vi "EXCOM_CRASH_TEST.vi"() -> ()   [LabVIEW 2011]
panel:
  in  "Infinite":bool
  out "TCP_string":string
  in  "offset DEC":dbl
  in  "offset RA":dbl
  in  "DEC (fix)":dbl format="%<%H:%M:%S%1u>t"
  in  "HA (fix)":dbl format="%<%H:%M:%S%1u>t"
  out "HA 2":dbl format="%.2f"
  out "DEC 2":dbl format="%.2f"
  out "NODEC":dbl format="%<%H:%M:%S%0u>t"
  out "NORA":dbl format="%<%H:%M:%S%1u>t"
  out "Epoque":dbl format="%.2f"
  out "DEC":dbl format="%<%H:%M:%S>t"
  out "RA":dbl format="%<%H:%M:%S%1u>t"
  out "HA":dbl format="%<%H:%M:%S%1u>t"
  out "Année":dbl format="%.2f"
  in  "Ring":u16(ring) items=["0 - No Command"=0, "1 - Update time and date"=1, "2 - ZDOMECOMMAND"=2, "3 - ZPOINT"=3, "4 - ZROTATOR"=4, "5 - ZFOCUS"=5, "6 - SLEW"=6, "7 - OFFSET"=7, "8 - OBJECT"=8, "9 - TMOVE"=9, "10 - ZENITH"=10, "11 - START TRAIL"=11, "12 - GO"=12, "13 - STOP"=13, "22 - DOEPOCH"=22, "36 - HA DEC SLEW"=36]
  out "STATLH":bool[](array[boolean])
  out "STATEX":bool[](array[boolean])
  in  "Délai de communication":u32(knob) scale=5.0..5000.0
  out "STATH":bool[](array[boolean])=[FALSE, FALSE, TRUE, TRUE, FALSE, TRUE, TRUE, FALSE, FALSE, FALSE, FALSE, FALSE, FALSE, FALSE, FALSE, FALSE, FALSE, FALSE, FALSE, FALSE, FALSE, FALSE, FALSE, FALSE, FALSE, FALSE, FALSE, FALSE, FALSE, FALSE, FALSE, FALSE]
  out "STATL":bool[](array[boolean])=[TRUE, FALSE, FALSE, FALSE, FALSE, FALSE, FALSE, FALSE, FALSE, FALSE, FALSE, FALSE, FALSE, FALSE, FALSE, FALSE, FALSE, FALSE, FALSE, FALSE, FALSE, FALSE, FALSE, FALSE, FALSE, FALSE, FALSE, FALSE, FALSE, FALSE, FALSE, FALSE]
  out "error out":errorcluster
  in  "QUITTER":bool
  out "connection ID":refnum<k5>
  # "."
  # "HA DEC ARGS"
  # "OFFSET ARGS"
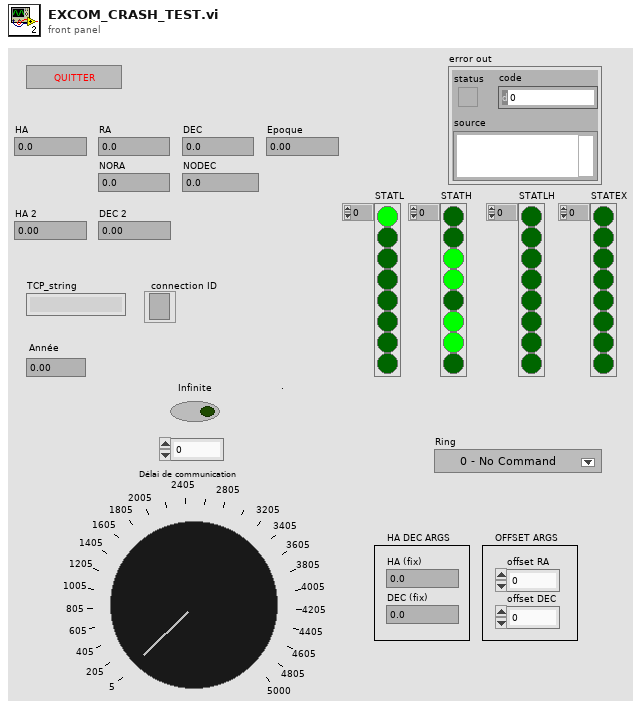
[diagram p1: front panel]
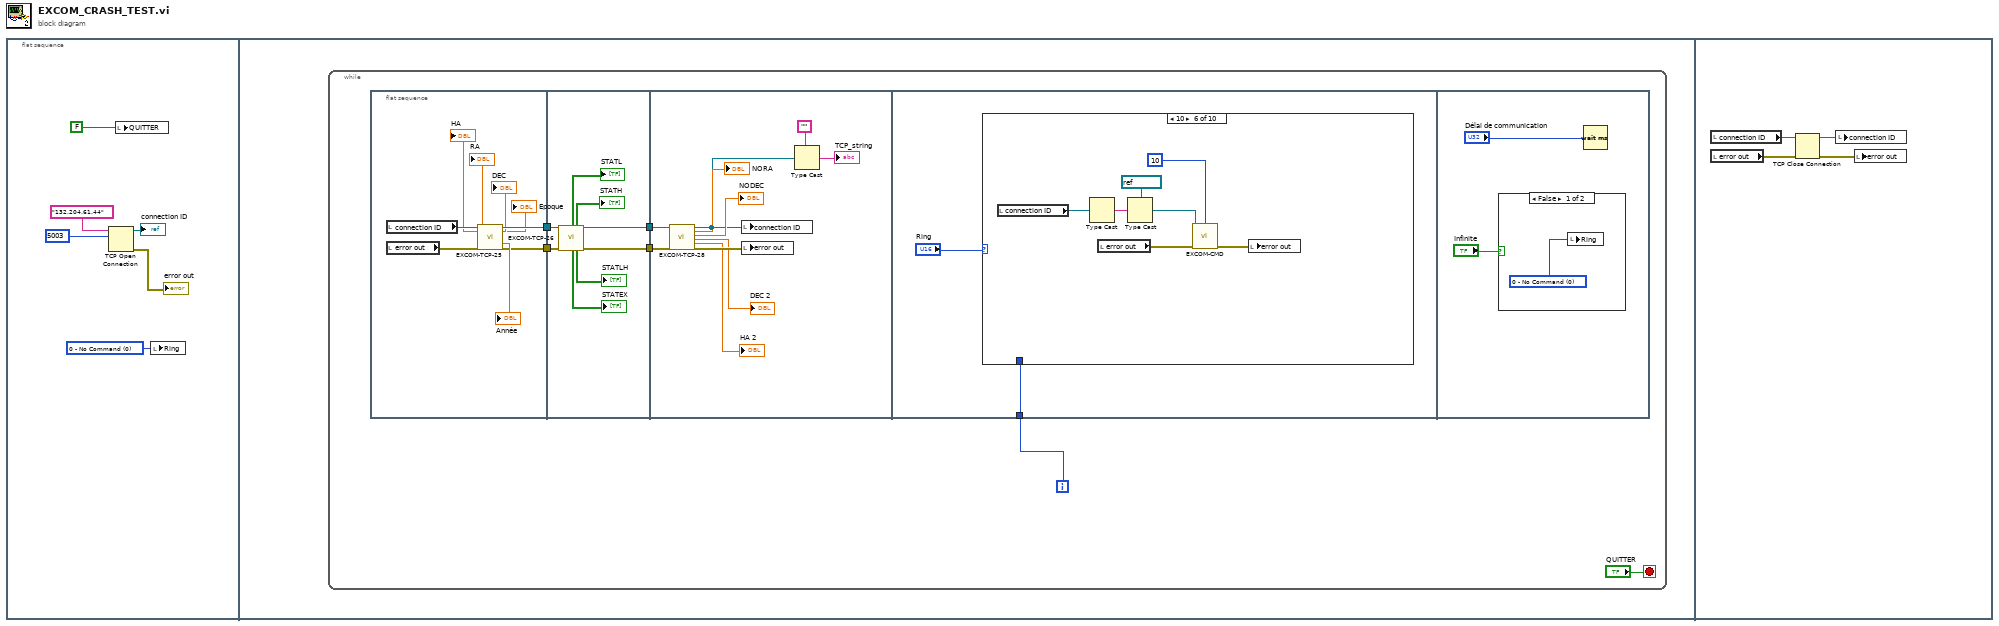
[diagram p0: block diagram]
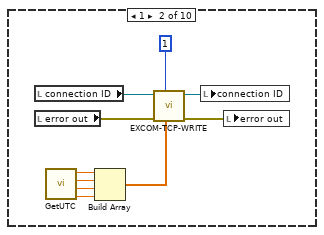
[diagram p3: hidden frame]
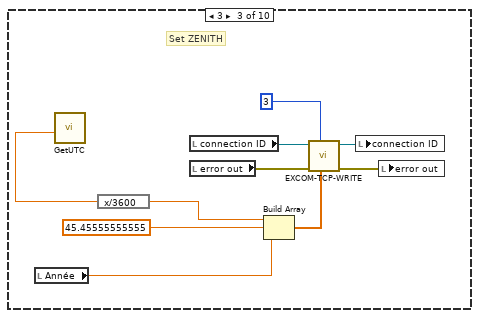
[diagram p4: hidden frame]
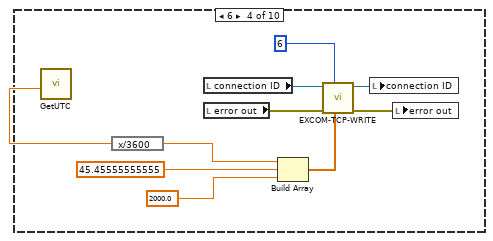
[diagram p5: hidden frame]
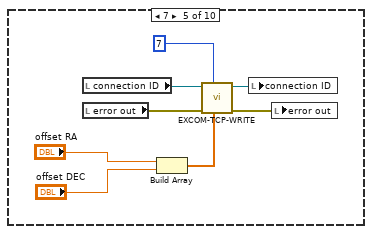
[diagram p6: hidden frame]
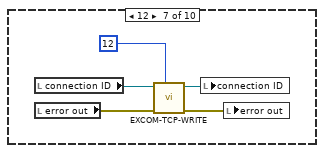
[diagram p7: hidden frame]
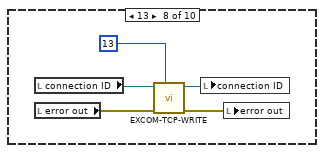
[diagram p8: hidden frame]
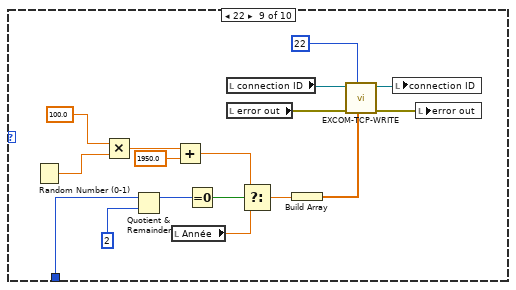
[diagram p9: hidden frame]
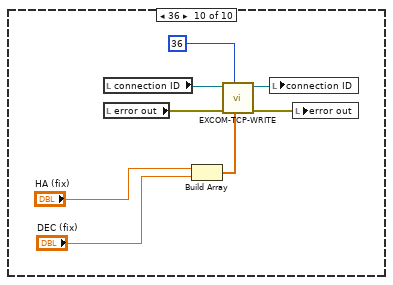
[diagram p10: hidden frame]
diagram:
  n1 = flat-sequence {
    frame #0 {
      w1 = u16 0 items=["0 - No Command"=0, "1 - Update time and date"=1, "2 - ZDOMECOMMAND"=2, "3 - ZPOINT"=3, "4 - ZROTATOR"=4, "5 - ZFOCUS"=5, "6 - SLEW"=6, "7 - OFFSET"=7, "8 - OBJECT"=8, "9 - TMOVE"=9, "10 - ZENITH"=10, "11 - START TRAIL"=11, "12 - GO"=12, "13 - STOP"=13, "22 - DOEPOCH"=22] ("Ring")
      n2 = TCP Open Connection(address="132.204.61.44", remote port or service name=u16 5003) -> (connection ID=→"connection ID":refnum<k5>, error out=→"error out":errorcluster)  [unwired: 3 in]
      n3 = local write "QUITTER"(FALSE ("QUITTER")) -> ()
      n4 = local write "Ring"(w1) -> ()
    }
    frame #1 {
      n5 = while {
        i -> [w11]
        stop <- "QUITTER" stop-if-true
        n6 = flat-sequence {
          tunnel: [w18] -> w10
          tunnel: [w17] -> w9
          tunnel: w10 -> [w24]
          tunnel: w9 -> [w25]
          tunnel: [w23] -> w8
          tunnel: [w22] -> w7
          tunnel: w8 -> [w39]
          tunnel: w7 -> [w38]
          tunnel: w11 -> [w40]
          frame #0 {
            n7 = local read "connection ID"() -> (w21:refnum<k5>)
            n8 = local read "error out"() -> (w20:errorcluster)
            n9 = call "EXCOM-TCP-25.vi"("connection ID"=w21, "Error IN"=w20) -> ("HA"=→"HA":dbl, "RA"=→"RA":dbl, "DEC"=→"DEC":dbl, "Epoque"=→"Epoque":dbl, "CID Out"=w18:refnum<k5>, "Année"=→"Année":dbl, "Error Out"=w17:errorcluster)  [unwired: 4 in, 7 out]
          }
          frame #1 {
            n10 = call "EXCOM-TCP-26.vi"("connection ID"=w24, "Error IN"=w25) -> ("STATL"=→"STATL":bool[], "STATH"=→"STATH":bool[], "CID Out"=w23:refnum<k5>, "STATEX"=→"STATEX":bool[], "STATLH"=→"STATLH":bool[], "Error Out"=w22:errorcluster)  [unwired: 8 in]
          }
          frame #2 {
            n11 = call "EXCOM-TCP-28.vi"("connection ID"=w39, "Error IN"=w38) -> ("CID Out"=w32:refnum<k5>, "NORA"=→"NORA":dbl, "NODEC"=→"NODEC":dbl, "DEC"=→"DEC 2":dbl, "HA"=→"HA 2":dbl, "Error Out"=w35:errorcluster)  [unwired: 12 in]
            n12 = local write "connection ID"(w32) -> ()
            n13 = local write "error out"(w35) -> ()
            n14 = Type Cast(type="", x=w32) -> (*(type *) &x=→"TCP_string":string)
          }
          frame #3 {
            n15 = case shown="10" "Ring" {
              tunnel: w40 -> [_ _ _ _ _ _ _ _ w103 _]
              frame 0, Default {
              }
              frame 1 {
                n16 = local read "connection ID"() -> (w51:refnum<k5>)
                n17 = local read "error out"() -> (w48:errorcluster)
                n18 = call "GetUTC.vi"() -> ("UTC_fractional"=w43:dbl, "Day"=w44:dbl, "Month"=w45:dbl, "Year"=w46:dbl)  [unwired: 5 out]
                n19 = Build Array(w46, w45, w44, w43) -> (w42:dbl[])
                n20 = call "EXCOM-TCP-WRITE.vi"("Args"=w42, "Commande #"=1, "Error IN"=w48, "connection ID"=w51) -> ("Error OUT"=w49:errorcluster, "connection ID out"=w50:refnum<k5>)  [unwired: 3 in, 2 out]
                n21 = local write "connection ID"(w50) -> ()
                n22 = local write "error out"(w49) -> ()
              }
              frame 3 {
                # "Set ZENITH"
                n23 = local read "Année"() -> (w52:dbl)
                n24 = call "GetUTC.vi"() -> ("LST+_seconds"=w53:dbl)  [unwired: 8 out]
                n25 = expression code="x/3600"(w53) -> (w55:dbl)
                n26 = local read "connection ID"() -> (w60:refnum<k5>)
                n27 = local read "error out"() -> (w57:errorcluster)
                n28 = Build Array(w55, 45.45555555555 ("element"), w52) -> (w56:dbl[])
                n29 = call "EXCOM-TCP-WRITE.vi"("Args"=w56, "Commande #"=3, "Error IN"=w57, "connection ID"=w60) -> ("Error OUT"=w58:errorcluster, "connection ID out"=w59:refnum<k5>)  [unwired: 3 in, 2 out]
                n30 = local write "connection ID"(w59) -> ()
                n31 = local write "error out"(w58) -> ()
              }
              frame 6 {
                n32 = call "GetUTC.vi"() -> ("LST+_seconds"=w63:dbl)  [unwired: 8 out]
                n33 = expression code="x/3600"(w63) -> (w64:dbl)
                n34 = local read "connection ID"() -> (w70:refnum<k5>)
                n35 = local read "error out"() -> (w67:errorcluster)
                n36 = Build Array(w64, 45.45555555555 ("element"), 2000.0 ("t")) -> (w66:dbl[])
                n37 = call "EXCOM-TCP-WRITE.vi"("Args"=w66, "Commande #"=6, "Error IN"=w67, "connection ID"=w70) -> ("Error OUT"=w68:errorcluster, "connection ID out"=w69:refnum<k5>)  [unwired: 3 in, 2 out]
                n38 = local write "connection ID"(w69) -> ()
                n39 = local write "error out"(w68) -> ()
              }
              frame 7 {
                n40 = local read "connection ID"() -> (w78:refnum<k5>)
                n41 = local read "error out"() -> (w75:errorcluster)
                n42 = Build Array("offset RA", "offset DEC") -> (w74:dbl[])
                n43 = call "EXCOM-TCP-WRITE.vi"("Args"=w74, "Commande #"=7, "Error IN"=w75, "connection ID"=w78) -> ("Error OUT"=w76:errorcluster, "connection ID out"=w77:refnum<k5>)  [unwired: 3 in, 2 out]
                n44 = local write "connection ID"(w77) -> ()
                n45 = local write "error out"(w76) -> ()
              }
              frame 10 {
                n46 = local read "connection ID"() -> (w81:refnum<k5>)
                n47 = Type Cast(x=w81) -> (*(type *) &x=w80:string)  [unwired: 1 in]
                n48 = local read "error out"() -> (w84:errorcluster)
                n49 = Type Cast(type=refnum<visa-resource-name> "ž \u0000\u0002" ("VRN OUT"), x=w80) -> (*(type *) &x=w83:refnum<visa-resource-name>)
                n50 = call "EXCOM-CMD.vi"("VRN IN"=w83, "Commande #"=10, "Error IN"=w84) -> ("Error OUT"=w85:errorcluster)  [unwired: 10 in, 2 out]
                n51 = local write "error out"(w85) -> ()
              }
              frame 12 {
                n52 = local read "connection ID"() -> (w90:refnum<k5>)
                n53 = local read "error out"() -> (w87:errorcluster)
                n54 = call "EXCOM-TCP-WRITE.vi"("Commande #"=12, "Error IN"=w87, "connection ID"=w90) -> ("Error OUT"=w88:errorcluster, "connection ID out"=w89:refnum<k5>)  [unwired: 4 in, 2 out]
                n55 = local write "connection ID"(w89) -> ()
                n56 = local write "error out"(w88) -> ()
              }
              frame 13 {
                n57 = local read "connection ID"() -> (w95:refnum<k5>)
                n58 = local read "error out"() -> (w92:errorcluster)
                n59 = call "EXCOM-TCP-WRITE.vi"("Commande #"=13, "Error IN"=w92, "connection ID"=w95) -> ("Error OUT"=w93:errorcluster, "connection ID out"=w94:refnum<k5>)  [unwired: 4 in, 2 out]
                n60 = local write "connection ID"(w94) -> ()
                n61 = local write "error out"(w93) -> ()
              }
              frame 22 {
                n62 = Random Number (0-1)() -> (number: 0 to 1=w102:dbl)
                n63 = Multiply(x=100.0, y=w102) -> (x*y=w100:dbl)
                n64 = Quotient & Remainder(x=w103, y=2) -> (x-y*floor(x/y)=w106:i32)  [unwired: 1 out]
                n65 = local read "Année"() -> (w98:dbl)
                n66 = Add(x=w100, y=1950.0) -> (x+y=w97:dbl)
                n67 = Equal To 0?(x=w106) -> (x = 0?=w107:bool)
                n68 = local read "connection ID"() -> (w112:refnum<k5>)
                n69 = local read "error out"() -> (w109:errorcluster)
                n70 = Select(t=w97, s=w107, f=w98) -> (s? t:f=w108:dbl)
                n71 = Build Array(w108) -> (w104:dbl[])
                n72 = call "EXCOM-TCP-WRITE.vi"("Args"=w104, "Commande #"=22, "Error IN"=w109, "connection ID"=w112) -> ("Error OUT"=w110:errorcluster, "connection ID out"=w111:refnum<k5>)  [unwired: 3 in, 2 out]
                n73 = local write "connection ID"(w111) -> ()
                n74 = local write "error out"(w110) -> ()
              }
              frame 36 {
                n75 = local read "connection ID"() -> (w120:refnum<k5>)
                n76 = local read "error out"() -> (w117:errorcluster)
                n77 = Build Array("HA (fix)", "DEC (fix)") -> (w116:dbl[])
                n78 = call "EXCOM-TCP-WRITE.vi"("Args"=w116, "Commande #"=36, "Error IN"=w117, "connection ID"=w120) -> ("Error OUT"=w118:errorcluster, "connection ID out"=w119:refnum<k5>)  [unwired: 3 in, 2 out]
                n79 = local write "connection ID"(w119) -> ()
                n80 = local write "error out"(w118) -> ()
              }
            }
          }
          frame #4 {
            n81 = case shown="False" "Infinite" {
              frame False {
                w124 = u16 0 items=["0 - No Command"=0, "1 - Update time and date"=1, "2 - ZDOMECOMMAND"=2, "3 - ZPOINT"=3, "4 - ZROTATOR"=4, "5 - ZFOCUS"=5, "6 - SLEW"=6, "7 - OFFSET"=7, "8 - OBJECT"=8, "9 - TMOVE"=9, "10 - ZENITH"=10, "11 - START TRAIL"=11, "12 - GO"=12, "13 - STOP"=13, "22 - DOEPOCH"=22, "36 - HA DEC SLEW"=36] ("Ring")
                n82 = local write "Ring"(w124) -> ()
              }
              frame True {
              }
            }
            n83 = Wait (ms)(milliseconds to wait="Délai de communication") -> ()  [unwired: 1 out]
          }
        }
      }
    }
    frame #2 {
      n84 = local read "connection ID"() -> (w128:refnum<k5>)
      n85 = local read "error out"() -> (w127:errorcluster)
      n86 = TCP Close Connection(connection ID=w128, error in (no error)=w127) -> (connection ID out=w125:refnum<k5>, error out=w126:errorcluster)  [unwired: 1 in]
      n87 = local write "connection ID"(w125) -> ()
      n88 = local write "error out"(w126) -> ()
    }
  }
